vi "Blacklist Connection.vi"(8 "error in (no error)":errorcluster, 9 "Channel 2":string, 10 "Channel 1":string, 11 "SLSC Switch in":refnum<class "SLSC Switch.lvclass">) -> (0 "error out":errorcluster, 1 "New Entry?":bool, 3 "SLSC Switch out":refnum<class "SLSC Switch.lvclass">)   [LabVIEW 2015, in "SLSC Switch.lvclass"]
uses:
  SLSC Switch.lvclass
  SLSC Switch.lvclass/SLSC Switch.ctl
  Controls/Connection.ctl
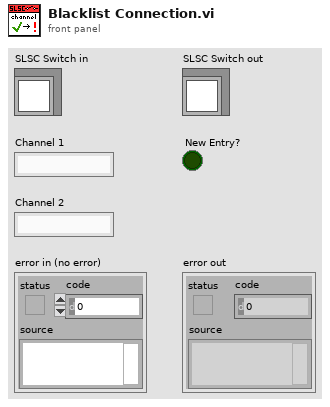
[diagram p1: front panel]
types:
  T1 = typedef "SLSC Switch.lvclass/Connection.ctl" = cluster{"channel 1":string, "channel 2":string}
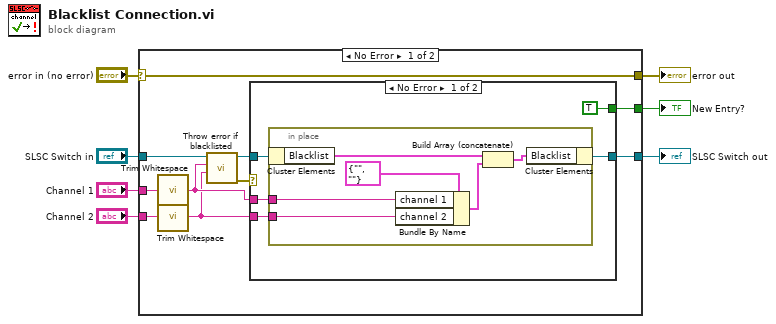
[diagram p0: block diagram]
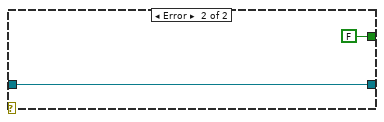
[diagram p2: hidden frame]
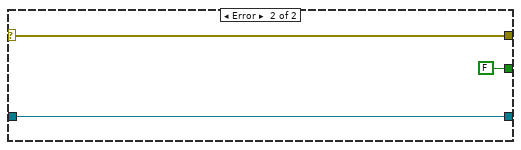
[diagram p3: hidden frame]
diagram:
  n1 = case shown="No Error" "error in (no error)" {
    selector: "error in (no error)" -> [w17 w33]
    tunnel: [w17 w33] -> w6
    tunnel: [w16 w32] -> w4
    tunnel: "SLSC Switch in" -> [w14 w32]
    tunnel: "Channel 1" -> [w11 _]
    tunnel: [w15 FALSE] -> w2
    tunnel: "Channel 2" -> [w10 _]
    frame No Error {
      n2 = call <vilib>:"Trim Whitespace.vi"("string"=w11) -> ("trimmed string"=w9:string)  [unwired: 1 in]
      n3 = call <vilib>:"Trim Whitespace.vi"("string"=w10) -> ("trimmed string"=w8:string)  [unwired: 1 in]
      n4 = call "Throw error if blacklisted.vi"("Channel 2"=w8, "Channel 1"=w9, "SLSC Switch in"=w14) -> ("error out"=w13:errorcluster, "SLSC Switch out"=w12:refnum<class "SLSC Switch.lvclass">)  [unwired: 6 in, 1 out]
      n5 = case shown="No Error" w13 {
        tunnel: [w22 w30] -> w16
        tunnel: [TRUE FALSE] -> w15
        tunnel: w12 -> [w21 w30]
        tunnel: w9 -> [w20 _]
        tunnel: w8 -> [w19 _]
        frame No Error {
          n6 = in-place {
            in-place-border: w20 -> [w26]
            in-place-border: w19 -> [w25]
            n7 = in-place-cluster #1(w21) -> ("Blacklist"=w28:T1[])
            n8 = Bundle By Name(cluster=T1 {"channel 1"="", "channel 2"=""} ("connections"), "channel 1"=w26, "channel 2"=w25) -> (w24:T1)
            n9 = Build Array (concatenate)(w28, w24) -> (w23:T1[])
            n10 = in-place-cluster #1("Blacklist"=w23) -> (w22:refnum<class "SLSC Switch.lvclass">)
          }
        }
        frame Error {
        }
      }
    }
    frame Error {
    }
  }
  "error out" <- w6
  "SLSC Switch out" <- w4
  "New Entry?" <- w2
